vi "Handle Listener Result.vi"(8 "error in (no error)":errorcluster, 10 "Result":T1, 11 "TCP Server in":refnum<class "TCP Server.lvclass">) -> (0 "error out":errorcluster, 1 "Send Ack":bool, 2 "Shutdown":bool, 3 "TCP Server out":refnum<class "TCP Server.lvclass">)   [LabVIEW 2020, in "Stream-TCP.lvlib" / "TCP Server.lvclass"]
uses:
  TCP Server.lvclass
  Listener Result.ctl
  TCP Client/TCP Client.lvclass
  Listener Status.ctl
  Stream-TCP.lvlib
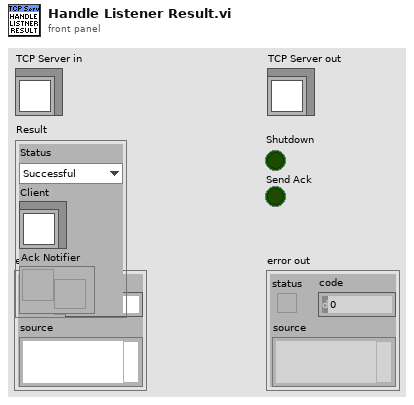
[diagram p1: front panel]
types:
  T1 = typedef "Stream-TCP.lvlib/Listener Result.ctl" = cluster{"Status":T2, "Client":refnum<class "TCP Client.lvclass">, "Ack Notifier":refnum<notifier>}
  T2 = typedef "Stream-TCP.lvlib/Listener Status.ctl" = enum16{"Successful", "Unsuccessful"}
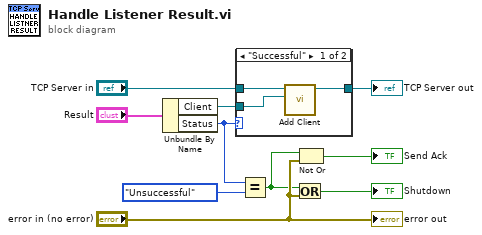
[diagram p0: block diagram]
diagram:
  n1 = Unbundle By Name("Result") -> ("Client"=w5:refnum<class "TCP Client.lvclass">, "Status"=w4:T2)
  n2 = case shown="\"Successful\"" w4 {
    tunnel: "TCP Server in" -> [w13 w14]
    tunnel: [w12 w14] -> w7
    tunnel: w5 -> [w11 _]
    frame "Successful" {
      n3 = call "Add Client.vi"("Client"=w11, "TCP Server in"=w13) -> ("TCP Server out"=w12:refnum<class "TCP Server.lvclass">)  [unwired: 8 in, 1 out]
    }
    frame "Unsuccessful" {
    }
  }
  "TCP Server out" <- w7
  n4 = Equal?(x=w4, y=Listener_Status."Unsuccessful") -> (x = y?=w2:bool)
  n5 = Or(x=w2, y="error in (no error)") -> (x .or. y?=→"Shutdown":bool)
  n6 = Not Or(1:"error in (no error)", 2:w2) -> (0:→"Send Ack":bool)
  "error out" <- "error in (no error)"
